vi "lvhttpd.vi"(7 "TCP Listen Port":u16=8080, 11 "Handlers":string[](array[string])=["Home", "Template", "File"]) -> ()   [LabVIEW 2011]
uses:
  tcp_client.ctl
  http_client.ctl
  http_request_response.ctl
  http_request.ctl
  http_field.ctl
  http_response.ctl
  template_field.ctl
  template_field_type.ctl
  <vilib>/Platform/TimedLoop/XDataNode/timing_clust.ctl
  <vilib>/Platform/TimedLoop/XDataNode/nitl_modes.ctl
  <vilib>/Platform/TimedLoop/XDataNode/wakeup.ctl
  <vilib>/Utility/error.llb/whitespace.ctl
  <vilib>/Platform/TimedLoop/XDataNode/XDataNode.xnode
  <vilib>/Platform/TimedLoop/XDataNode/XDNodeRunTimeDep.lvlib
  <vilib>/NI_Real-Time Target Support.lvlib
panel:
  in  "stop server":bool
  out "String":string
  # "lvhttpd - LabView HTTP Web Server"
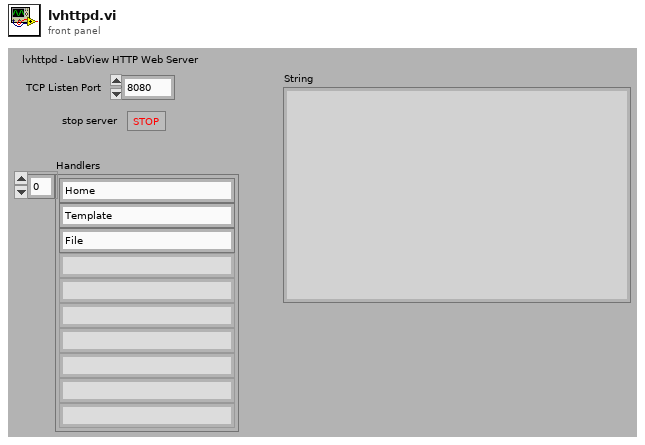
[diagram p1: front panel]
types:
  T1 = typedef "http_client.ctl" = cluster{"connection":refnum<k5>, "buffer":string, "HTTP Request":T2}
  T2 = typedef "http_request_response.ctl" = cluster{"Request":T3, "Request Header Fields":T4[], "Response Header Fields":T4[], "Request Message body":string, "Response Message body":string, "Response":T5, "Template":string, "Template Fields":T6[]}
  T3 = typedef "http_request.ctl" = cluster{"Method":string, "Resource":string, "Protocol":string}
  T4 = typedef "http_field.ctl" = cluster{"Field":string, "Value":string}
  T5 = typedef "http_response.ctl" = cluster{"Protocol":string, "Status code":dbl, "Description":string}
  T6 = typedef "template_field.ctl" = cluster{"Name":string, "Template Field Type":T7, "data":variant}
  T7 = typedef "template_field_type.ctl" = enum16{"string", "string array", "number", "number array", "cluster", "cluster array"}
  T8 = typedef "tcp_client.ctl" = cluster{"connection ID":refnum<k5>, "Buffer":string, "Remote adress":string, "accessed last time at":timestamp}
  T9 = typedef "XDNodeRunTimeDep.lvlib/timing_clust.ctl" = cluster{"Expected End [f-1]":u64, "Actual End [f-1]":u64, "Finished Late? [f-1]":bool, "Expected End [i-1]":u64, "Actual End [i-1]":u64, "Finished Late? [i-1]":bool, "Expected Start [i]":u64, "Actual Start [i]":u64, "Expected Start [f]":u64, "Actual Start [f]":u64, "Source Name":string, "Structure Name":string, "Period":i64, "Deadline":i64, "Offset":i64, "Start":i64, "Priority":i32, "Timeout":i32, "Mode":T10, "Wakeup Reason":T11, "Error":errorcluster, "Source Type":string, "Secondary Source Type":string, "Global End Time":u64, "Global Start Time":u64, "Frame Duration":u64, "Iteration Duration":u64, "Assigned CPU":i32, "I/O Scan Engine Mode":u32}
  T10 = typedef "XDNodeRunTimeDep.lvlib/nitl_modes.ctl" = enum32{"No Change", "Process missed periods, maintain original phase", "Discard missed periods, maintain original phase", "Process missed periods, ignore original phase", "Discard missed periods, ignore original phase"}
  T11 = typedef "XDNodeRunTimeDep.lvlib/wakeup.ctl" = enum32{"Normal", "Aborted", "Asynchronous wakeup", "Timing source error", "Timed loop error", "Timeout"}
  T12 = enum16{"Standard", "Buffered", "CRLF", "Immediate"}
  T13 = typedef "whitespace.ctl" = u16
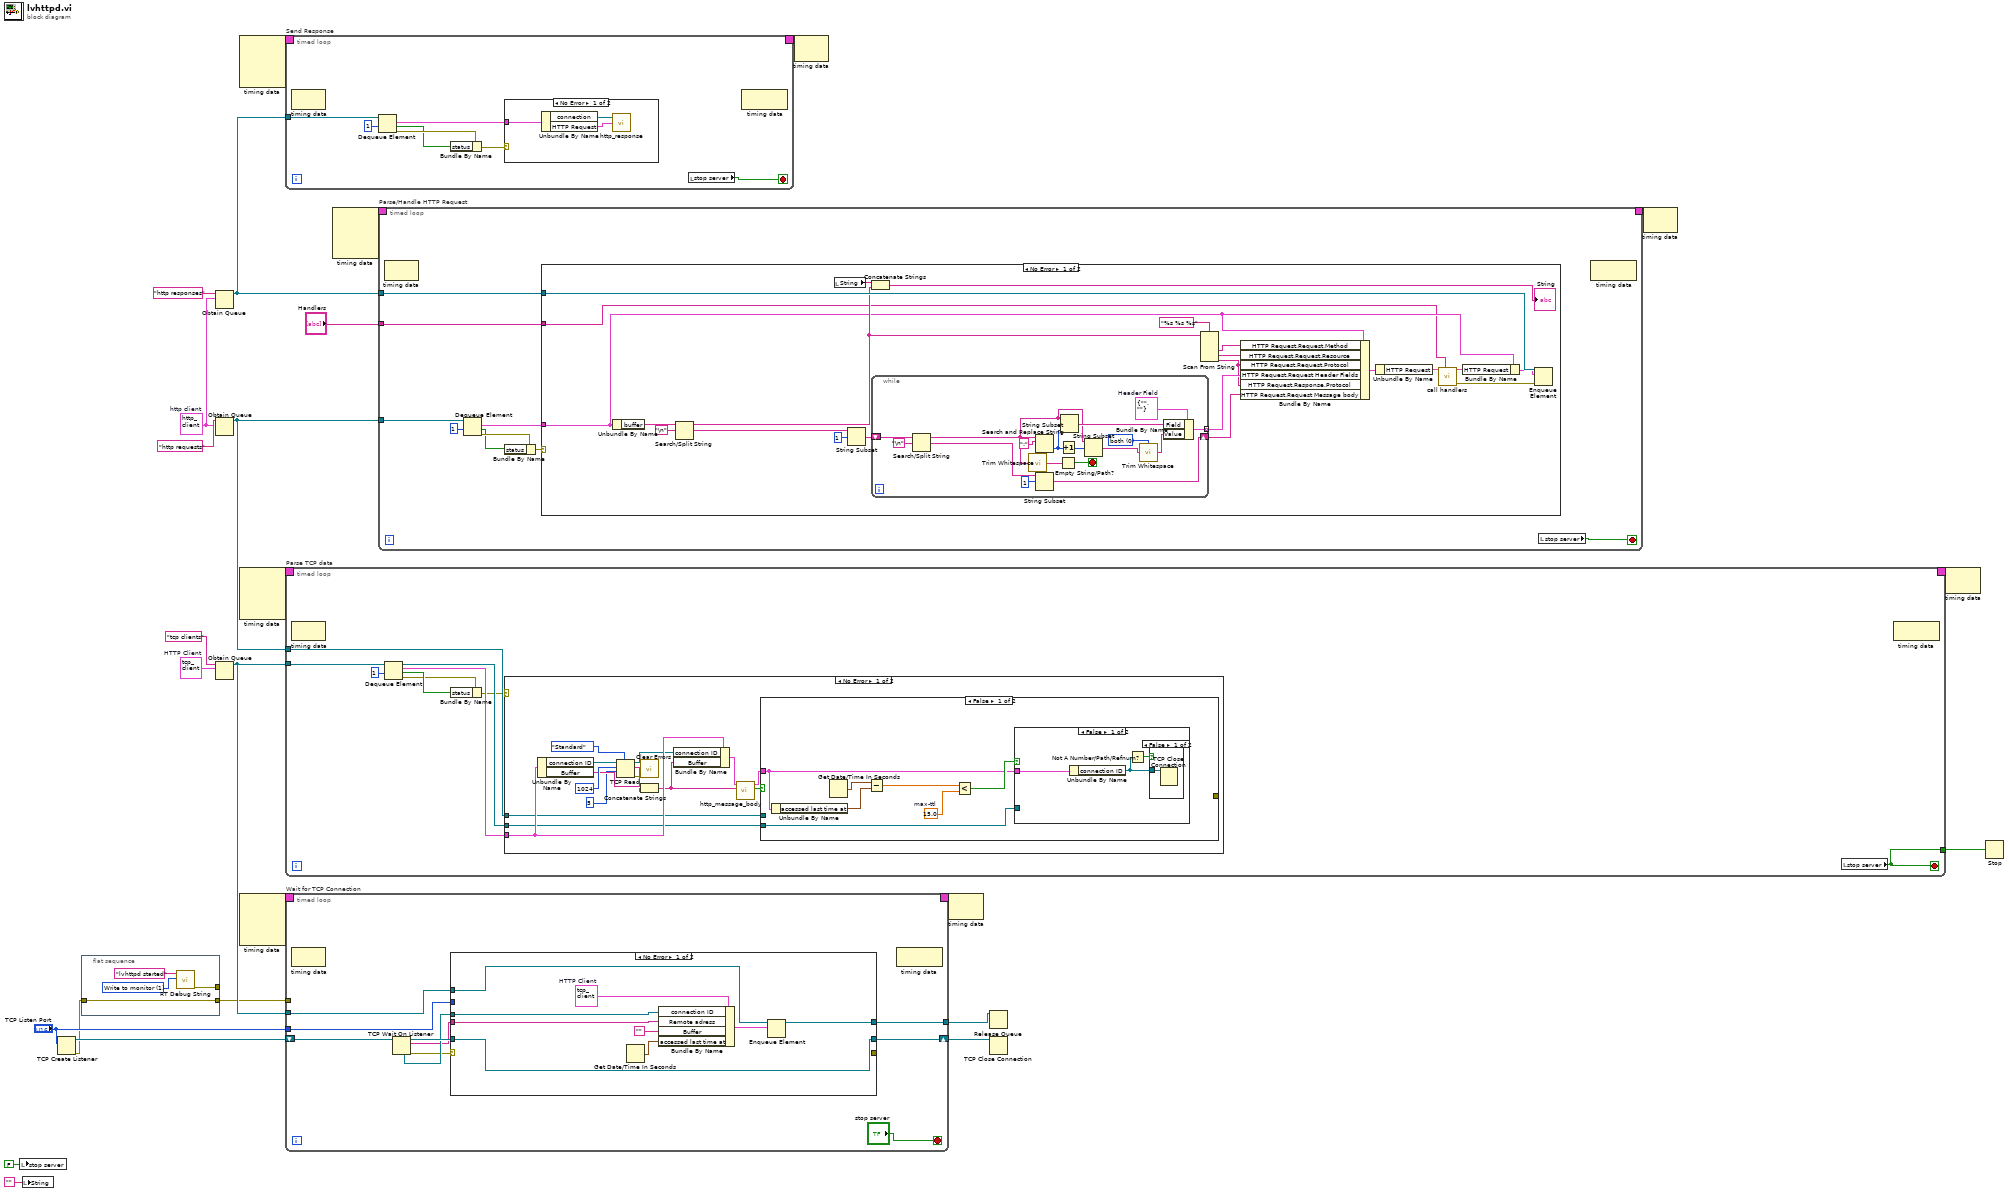
[diagram p0: block diagram]
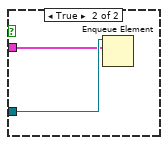
[diagram p3: hidden frame]
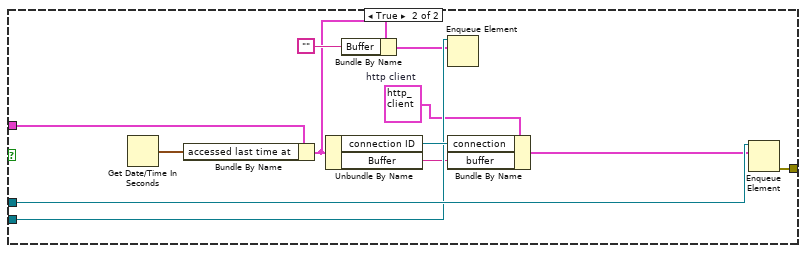
[diagram p4: hidden frame]
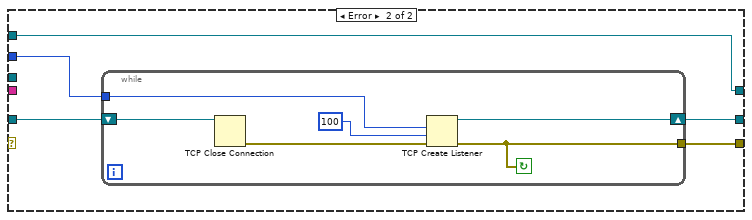
[diagram p6: hidden frame]
diagram:
  w18 = T1 {"connection"=refnum, "buffer"="", "HTTP Request"={"Request"={"Method"="", "Resource"="", "Protocol"=""}, "Request Header Fields"=[], "Response Header Fields"=[], "Request Message body"="", "Response Message body"="", "Response"={"Protocol"="", "Status code"=0.0, "Description"=""}, "Template"="", "Template Fields"=[]}}  # http client
  w21 = T8 {"connection ID"=refnum, "Buffer"="", "Remote adress"="", "accessed last time at"=timestamp(0 s since 1904-01-01)}  # HTTP Client
  n1 = local write "stop server"(FALSE ("stop server")) -> ()
  n2 = local write "String"("") -> ()
  n3 = TCP Create Listener(10:"TCP Listen Port") -> (0:w3:errorcluster, 3:w26:refnum<k5>)  [unwired: 4 in, 1 out]
  n4 = flat-sequence {
    tunnel: w3 -> [w30]
    tunnel: [w30] -> w2
    tunnel: [w28] -> _
    frame #0 {
      w27 = u16 1 items=["Write to serial", "Write to monitor"] ("Interface")
      n5 = call <vilib>:"RT Debug String.vi"("Interface"=w27, "String to write"="lvhttpd started") -> ("error out"=w28:errorcluster)  [unwired: 9 in]
    }
  }
  n6 = Obtain Queue(name (unnamed)="http responses", element data type=w18) -> (queue out=w16:refnum<queue>)  [unwired: 3 in, 2 out]
  n7 = Obtain Queue(name (unnamed)="http requests", element data type=w18) -> (queue out=w19:refnum<queue>)  [unwired: 3 in, 2 out]
  n8 = Obtain Queue(name (unnamed)="tcp clients", element data type=w21) -> (queue out=w22:refnum<queue>)  [unwired: 3 in, 2 out]
  n9 = node-c288() -> (w11:T9)  [unwired: 4 in]
  n10 = node-c288() -> (w5:T9)  [unwired: 4 in]
  n11 = node-c288() -> (w7:T9)  [unwired: 4 in]
  n12 = timed-loop "Send Response" {
    tunnel: w16 -> [w37]
    timing: w11 -> [_]
    timing-out: [_] -> w10
    stop <- w35 stop-if-true
    n13 = node-c288() -> ()  [unwired: 1 in, 1 out]
    n14 = Dequeue Element(queue=w37, timeout in ms (-1)=1) -> (element=w36:T1, timed out?=w31:bool, error out=w33:errorcluster)  [unwired: 1 in, 1 out]
    n15 = Bundle By Name(cluster=w33, "status"=w31) -> (w32:errorcluster)
    n16 = case shown="No Error" w32 {
      tunnel: w36 -> [w42 _]
      frame No Error {
        n17 = Unbundle By Name(w42) -> ("connection"=w41:refnum<k5>, "HTTP Request"=w40:T2)
        n18 = call "http_response.vi"("HTTP Request"=w40, "listener ID"=w41) -> ()  [unwired: 1 in, 3 out]
      }
      frame Error {
      }
    }
    n19 = local read "stop server"() -> (w35:bool)
    n20 = node-c288() -> ()  [unwired: 1 in, 1 out]
  }
  n21 = timed-loop "Parse TCP data" {
    tunnel: w22 -> [w51]
    tunnel: w19 -> [w48]
    tunnel: [w43] -> w12
    timing: w5 -> [_]
    timing-out: [_] -> w4
    stop <- w43 stop-if-true
    n22 = node-c288() -> ()  [unwired: 1 in, 1 out]
    n23 = Dequeue Element(queue=w51, timeout in ms (-1)=1) -> (queue out=w49:refnum<queue>, element=w50:T8, timed out?=w46:bool, error out=w45:errorcluster)  [unwired: 1 in]
    n24 = Bundle By Name(cluster=w45, "status"=w46) -> (w44:errorcluster)
    n25 = case shown="No Error" w44 {
      tunnel: w50 -> [w66 _]
      tunnel: w49 -> [w65 _]
      tunnel: w48 -> [w63 _]
      frame No Error {
        n26 = Unbundle By Name(w66) -> ("connection ID"=w68:refnum<k5>, "Buffer"=w61:string)
        n27 = TCP Read(connection ID=w68, bytes to read=1024, 7:T12."Standard" ("mode (standard)"), 9:5 ("timeout ms (25000)")) -> (connection ID out=w64:refnum<k5>, data out=w60:string, error out=w58:errorcluster)  [unwired: 1 in]
        n28 = call <vilib>:"Clear Errors.vi"("error in (no error)"=w58) -> ()  [unwired: 6 in, 1 out]
        n29 = Concatenate Strings(w61, w60) -> (w54:string)
        n30 = Bundle By Name(cluster=w66, "connection ID"=w64, "Buffer"=w54) -> (w56:T8)
        n31 = call "http_message_body.vi"("String"=w54, "HTTP Client in"=w56) -> ("Boolean"=w57:bool, "HTTP Client out"=w55:T8)  [unwired: 8 in]
        n32 = case shown="False" w57 {
          tunnel: w65 -> [w70 w91]
          tunnel: w55 -> [w69 w90]
          tunnel: w63 -> [_ w93]
          tunnel: [_ w82] -> _
          frame False {
            w72 = 15.0  # max-ttl
            n33 = Unbundle By Name(w69) -> ("accessed last time at"=w74:timestamp)
            n34 = Get Date/Time In Seconds() -> (seconds since 1Jan1904=w75:timestamp)
            n35 = Subtract(x=w75, y=w74) -> (x-y=w73:dbl)
            n36 = Less?(x=w73, y=w72) -> (x < y?=w71:bool)
            n37 = case shown="False" w71 {
              tunnel: w70 -> [_ w81]
              tunnel: w69 -> [w78 w80]
              frame False {
                n38 = Unbundle By Name(w78) -> ("connection ID"=w77:refnum<k5>)
                n39 = Not A Number/Path/Refnum?(number/path/refnum=w77) -> (NaN/Path/Refnum?=w76:bool)
                n40 = case shown="False" w76 {
                  tunnel: w77 -> [w79 _]
                  frame False {
                    n41 = TCP Close Connection(connection ID=w79) -> ()  [unwired: 2 in, 2 out]
                  }
                  frame True {
                  }
                }
              }
              frame True {
                n42 = Enqueue Element(queue=w81, element=w80) -> ()  [unwired: 2 in, 3 out]
              }
            }
          }
          frame True {
            w89 = T1 {"connection"=refnum, "buffer"="", "HTTP Request"={"Request"={"Method"="", "Resource"="", "Protocol"=""}, "Request Header Fields"=[], "Response Header Fields"=[], "Request Message body"="", "Response Message body"="", "Response"={"Protocol"="", "Status code"=0.0, "Description"=""}, "Template"="", "Template Fields"=[]}}  # http client
            n43 = Get Date/Time In Seconds() -> (seconds since 1Jan1904=w83:timestamp)
            n44 = Bundle By Name(cluster=w90, "accessed last time at"=w83) -> (w84:T8)
            n45 = Unbundle By Name(w84) -> ("connection ID"=w92:refnum<k5>, "Buffer"=w87:string)
            n46 = Bundle By Name(cluster=w84, "Buffer"="") -> (w86:T8)
            n47 = Enqueue Element(queue=w91, element=w86) -> ()  [unwired: 2 in, 3 out]
            n48 = Bundle By Name(cluster=w89, "connection"=w92, "buffer"=w87) -> (w88:T1)
            n49 = Enqueue Element(queue=w93, element=w88) -> (error out=w82:errorcluster)  [unwired: 2 in, 2 out]
          }
        }
      }
      frame Error {
      }
    }
    n50 = local read "stop server"() -> (w43:bool)
    n51 = node-c288() -> ()  [unwired: 1 in, 1 out]
  }
  n52 = timed-loop "Wait for TCP Connection" {
    shift-right: [w102] -> w25
    shift-left: w26 -> [w103]
    tunnel: "TCP Listen Port" -> [w100]
    tunnel: w22 -> [w96]
    tunnel: [w95] -> w23
    timing: w7 -> [_]
    timing-out: [_] -> w6
    tunnel: w2 -> [_]
    stop <- "stop server" stop-if-true
    n53 = node-c288() -> ()  [unwired: 1 in, 1 out]
    n54 = TCP Wait On Listener(11:w103) -> (0:w94:errorcluster, 2:w97:string, 3:w101:refnum<k5>, 4:w98:refnum<k5>)  [unwired: 3 in, 1 out]
    n55 = case shown="No Error" w94 {
      tunnel: [w114 w117] -> w102
      tunnel: w101 -> [w114 w119]
      tunnel: w100 -> [_ w118]
      tunnel: w98 -> [w112 _]
      tunnel: w97 -> [w111 _]
      tunnel: w96 -> [w109 w116]
      tunnel: [w107 w116] -> w95
      tunnel: [_ w115] -> _
      frame No Error {
        w113 = T8 {"connection ID"=refnum, "Buffer"="", "Remote adress"="", "accessed last time at"=timestamp(0 s since 1904-01-01)}  # HTTP Client
        n56 = Get Date/Time In Seconds() -> (seconds since 1Jan1904=w106:timestamp)
        n57 = Bundle By Name(cluster=w113, "connection ID"=w112, "Remote adress"=w111, "Buffer"="", "accessed last time at"=w106) -> (w108:T8)
        n58 = Enqueue Element(queue=w109, element=w108) -> (queue out=w107:refnum<queue>)  [unwired: 2 in, 2 out]
      }
      frame Error {
        n59 = while {
          tunnel: w118 -> [w124]
          tunnel: [w120] -> w115
          shift-right: [w122] -> w117
          shift-left: w119 -> [w125]
          stop <- w120 continue-if-true
          n60 = TCP Close Connection(connection ID=w125) -> (error out=w123:errorcluster)  [unwired: 2 in, 1 out]
          n61 = TCP Create Listener(8:w123, 9:100 ("timeout ms (25000)"), 10:w124) -> (0:w120:errorcluster, 3:w122:refnum<k5>)  [unwired: 2 in, 1 out]
        }
      }
    }
    n62 = node-c288() -> ()  [unwired: 1 in, 1 out]
  }
  n63 = node-c288() -> (w9:T9)  [unwired: 4 in]
  n64 = timed-loop "Parse/Handle HTTP Request" {
    tunnel: w19 -> [w134]
    tunnel: w16 -> [w133]
    timing: w9 -> [_]
    timing-out: [_] -> w8
    tunnel: "Handlers" -> [w126]
    stop <- w131 stop-if-true
    n65 = node-c288() -> ()  [unwired: 1 in, 1 out]
    n66 = Dequeue Element(queue=w134, timeout in ms (-1)=1) -> (element=w132:T1, timed out?=w127:bool, error out=w129:errorcluster)  [unwired: 1 in, 1 out]
    n67 = Bundle By Name(cluster=w129, "status"=w127) -> (w128:errorcluster)
    n68 = case shown="No Error" w128 {
      tunnel: w133 -> [w153 _]
      tunnel: w132 -> [w143 _]
      tunnel: w126 -> [w137 _]
      frame No Error {
        n69 = Unbundle By Name(w143) -> ("buffer"=w149:string)
        n70 = Search/Split String(string=w149, search string/char (-)="\n") -> (substring before match=w144:string, match + rest of string=w151:string)  [unwired: 1 in, 1 out]
        n71 = local read "String"() -> (w146:string)
        n72 = String Subset(string=w151, offset (0)=1) -> (substring=w148:string)  [unwired: 1 in]
        n73 = Concatenate Strings(w146, w144) -> (→"String":string)
        n74 = while {
          tunnel: [w172] -> w155 mode=indexing
          shift-right: [w167] -> w141
          shift-left: w148 -> [w165]
          stop <- w164 stop-if-true
          w175 = T13 0 items=["both", "start of string", "end of string"] ("location (both)")
          w173 = T4 {"Field"="", "Value"=""}  # Header Field
          n75 = Search/Split String(string=w165, search string/char (-)="\n") -> (substring before match=w160:string, match + rest of string=w166:string)  [unwired: 1 in, 1 out]
          n76 = call <vilib>:"Trim Whitespace.vi"("string"=w160) -> ("trimmed string"=w161:string)  [unwired: 1 in]
          n77 = String Subset(string=w166, offset (0)=1) -> (substring=w167:string)  [unwired: 1 in]
          n78 = Search and Replace String(input string=w160, search string=":") -> (offset past replacement=w162:i32)  [unwired: 6 in, 3 out]
          n79 = Empty String/Path?(string/path=w161) -> (empty?=w164:bool)
          n80 = Increment(x=w162) -> (x+1=w159:i32)
          n81 = String Subset(string=w160, length (rest)=w162) -> (substring=w163:string)  [unwired: 1 in]
          n82 = String Subset(string=w160, offset (0)=w159) -> (substring=w170:string)  [unwired: 1 in]
          n83 = call <vilib>:"Trim Whitespace.vi"("string"=w170, "location (both)"=w175) -> ("trimmed string"=w174:string)
          n84 = Bundle By Name(cluster=w173, "Field"=w163, "Value"=w174) -> (w172:T4)
        }
        n85 = Scan From String(format string="%s %s %s", input string=w144) -> (output 1=w157:string, output 2=w158:string, output 3=w142:string)  [unwired: 5 in, 3 out]
        n86 = Bundle By Name(cluster=w143, "HTTP Request.Request.Method"=w157, "HTTP Request.Request.Resource"=w158, "HTTP Request.Request.Protocol"=w142, "HTTP Request.Request Header Fields"=w155, "HTTP Request.Response.Protocol"=w142, "HTTP Request.Request Message body"=w141) -> (w154:T1)
        n87 = Unbundle By Name(w154) -> ("HTTP Request"=w140:T2)
        n88 = call "call handlers.vi"("Handlers"=w137, "HTTP Request in"=w140) -> ("error out"=w138:errorcluster, "HTTP Request out"=w139:T2)  [unwired: 7 in, 1 out]
        n89 = Bundle By Name(cluster=w143, "HTTP Request"=w139) -> (w152:T1)
        n90 = Enqueue Element(queue=w153, element=w152, error in (no error)=w138) -> ()  [unwired: 1 in, 3 out]
      }
      frame Error {
      }
    }
    n91 = local read "stop server"() -> (w131:bool)
    n92 = node-c288() -> ()  [unwired: 1 in, 1 out]
  }
  n93 = node-c288(w10) -> ()  [unwired: 1 out]
  n94 = node-c288(w6) -> ()  [unwired: 1 out]
  n95 = Release Queue(queue=w23) -> ()  [unwired: 2 in, 3 out]
  n96 = TCP Close Connection(connection ID=w25) -> ()  [unwired: 2 in, 2 out]
  n97 = node-c288(w8) -> ()  [unwired: 1 out]
  n98 = node-c288(w4) -> ()  [unwired: 1 out]
  n99 = Stop(stop? (T)=w12) -> ()
